vi "Oscillate.vi"(0 "controller in":refnum<k24>, 1 "Cycles":i32, 2 "NumFreqs":i32, 5 "Distance":dbl, 7 "Frequency":dbl, 9 "axis name":string, 11 "error in (no error)":errorcluster, 12 "taskId":i32(ring) items=["TLibrary", "T01", "T02", "T03", "T04", "T05", "T06", "T07", "T08", "T09", "T10", "T11", "T12", "T13", "T14", "T15", "T16", "T17", "T18", "T19", "T20", "T21", "T22", "T23", "T24", "T25", "T26", "T27", "T28", "T29", "T30", "T31"]) -> (4 "controller out":refnum<k24>, 15 "error out":errorcluster)   [LabVIEW 2021]
uses:
  C:/Program Files (x86)/Aerotech/A3200/LabVIEW/2010/Bin/Aerotech.A3200.dll
  Bin/Aerotech.A3200.dll
  C:/Program Files (x86)/Aerotech/A3200/LabVIEW/2010/Bin/Aerotech.A3200.LabVIEW.dll
  Bin/Aerotech.A3200.LabVIEW.dll
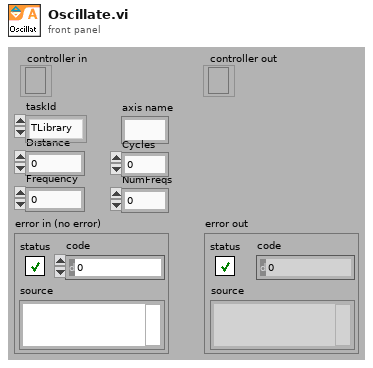
[diagram p1: front panel]
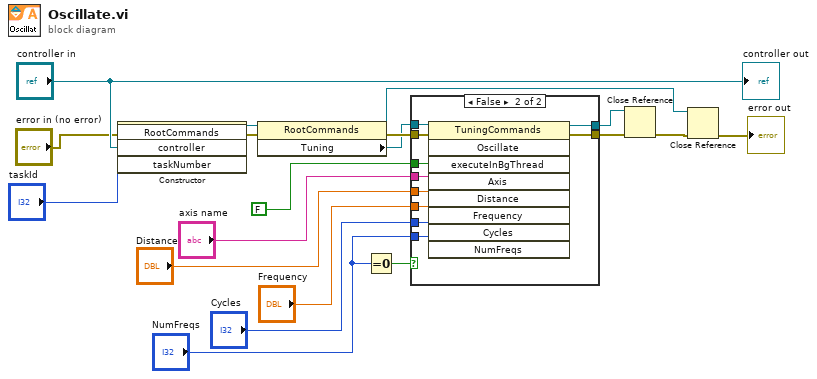
[diagram p0: block diagram]
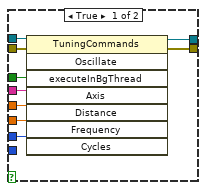
[diagram p2: hidden frame]
diagram:
  n1 = constructor class="RootCommands"(error in="error in (no error)", "controller"="controller in", "taskNumber"="taskId") -> (reference out=w9:refnum<k24>, error out=w10:errorcluster)  [unwired: 2 in, 3 out]
  n2 = property class="RootCommands"(reference=w9, error in=w10) -> (reference out=w14:refnum<k24>, error out=w8:errorcluster, "Tuning"=w7:refnum<k24>)
  n3 = Equal To 0?(x="NumFreqs") -> (x = 0?=w3:bool)
  n4 = case shown="False" w3 {
    tunnel: [w28 w36] -> w12
    tunnel: [w27 w35] -> w11
    tunnel: w8 -> [w26 w38]
    tunnel: w7 -> [w25 w37]
    tunnel: "NumFreqs" -> [_ w34]
    tunnel: "axis name" -> [w24 w32]
    tunnel: "Distance" -> [w23 w33]
    tunnel: FALSE ("return immediately") -> [w22 w31]
    tunnel: "Frequency" -> [w20 w30]
    tunnel: "Cycles" -> [w21 w29]
    frame True {
      n5 = invoke class="TuningCommands" method="Oscillate"(reference=w25, error in=w26, "executeInBgThread"=w22, "Axis"=w24, "Distance"=w23, "Frequency"=w20, "Cycles"=w21) -> (reference out=w28:refnum<k24>, error out=w27:errorcluster)  [unwired: 1 in, 6 out]
    }
    frame False {
      n6 = invoke class="TuningCommands" method="Oscillate"(reference=w37, error in=w38, "executeInBgThread"=w31, "Axis"=w32, "Distance"=w33, "Frequency"=w30, "Cycles"=w29, "NumFreqs"=w34) -> (reference out=w36:refnum<k24>, error out=w35:errorcluster)  [unwired: 1 in, 7 out]
    }
  }
  n7 = Close Reference(reference=w12, error in (no error)=w11) -> (error out=w13:errorcluster)
  n8 = Close Reference(reference=w14, error in (no error)=w13) -> (error out=→"error out":errorcluster)
  "controller out" <- "controller in"
